vi "HEWH Find Draw Start.vi"(8 "Error In":errorcluster, 10 "End of First Draw":i32, 11 "Array":string[][](array[string])) -> (0 "Error Out":errorcluster, 2 "Draw Start":i32)   [LabVIEW 2016]
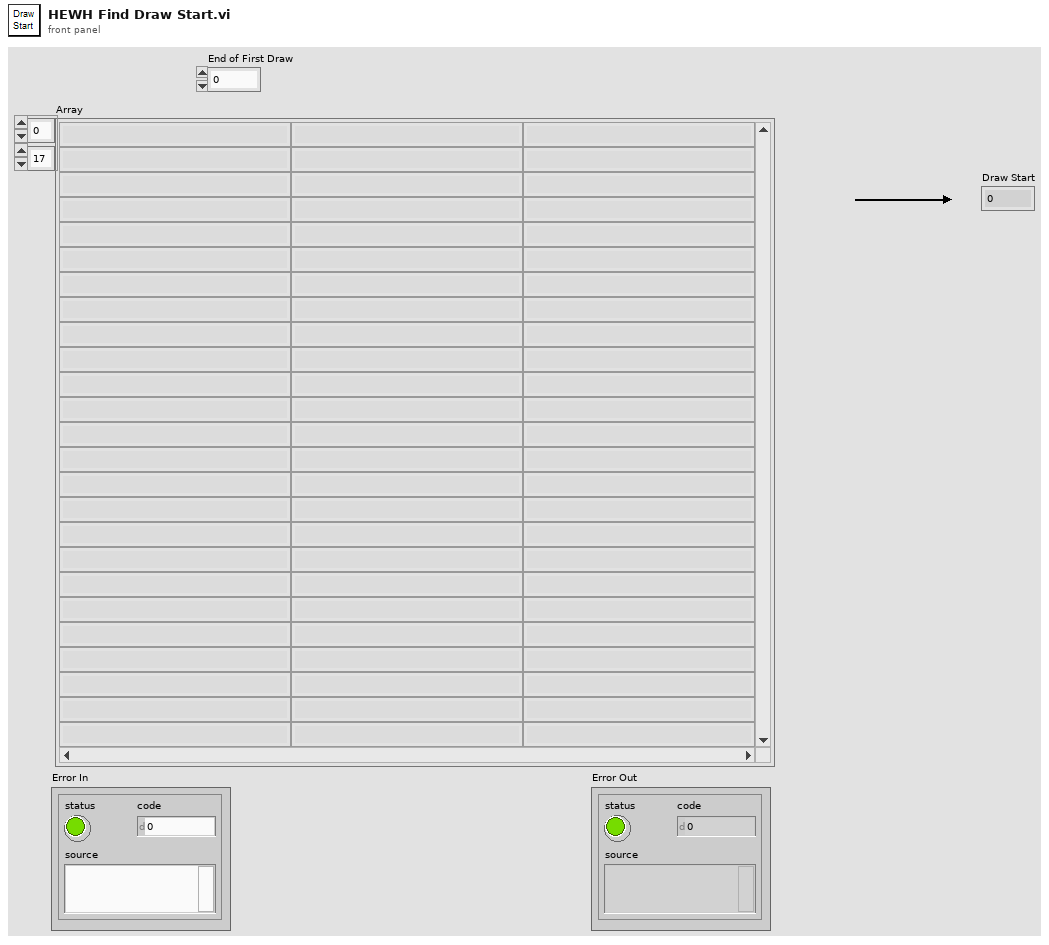
[diagram p1: front panel]
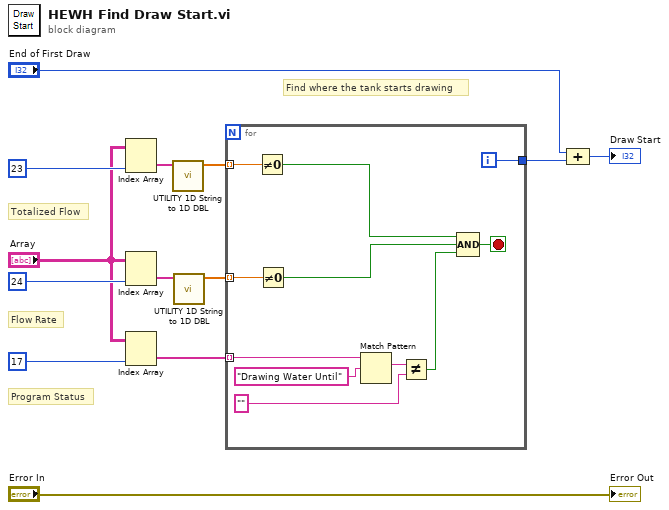
[diagram p0: block diagram]
diagram:
  # "Totalized Flow"
  # "Find where the tank starts drawing"
  # "Program Status"
  # "Flow Rate"
  n1 = Index Array(array="Array", index (col)=23 ("disabled index (col)")) -> (element=w3:string[])  [unwired: 1 in]
  n2 = Index Array(array="Array", index (col)=24 ("disabled index (col)")) -> (element=w4:string[])  [unwired: 1 in]
  n3 = Index Array(array="Array", index (col)=17 ("disabled index (col)")) -> (element=w12:string[])  [unwired: 1 in]
  n4 = call "UTILITY 1D String to 1D DBL.vi"("Save Data"=w3) -> ("DBL"=w2:dbl[])  [unwired: 10 in]
  n5 = call "UTILITY 1D String to 1D DBL.vi"("Save Data"=w4) -> ("DBL"=w1:dbl[])  [unwired: 10 in]
  n6 = for {
    tunnel: w12 -> [w24] mode=indexing
    tunnel: [w21] -> w5
    tunnel: w2 -> [w19] mode=indexing
    tunnel: w1 -> [w18] mode=indexing
    i -> [w21]
    stop <- w15 stop-if-true
    n7 = Not Equal To 0?(x=w19) -> (x != 0?=w16:bool)
    n8 = Not Equal To 0?(x=w18) -> (x != 0?=w17:bool)
    n9 = Match Pattern(string=w24, regular expression="Drawing Water Until") -> (match substring=w20:string)  [unwired: 1 in, 3 out]
    n10 = Not Equal?(x=w20, y="") -> (x != y?=w14:bool)
    n11 = Compound Arithmetic op=AND(w16, w17, w14) -> (w15:bool)
  }
  n12 = Compound Arithmetic op=ADD("End of First Draw", w5) -> (→"Draw Start":i32)
  "Error Out" <- "Error In"
